vi "Reset Progress.vi"(8 "error in (no error)":errorcluster {"code" format="Error %.0f"}, 11 "UI Interaction in":refnum<class "UI Interaction.lvclass">) -> (0 "error out":errorcluster {"code" format="Error %.0f"}, 3 "UI Interaction out":refnum<class "UI Interaction.lvclass">)   [LabVIEW 2023, in "UI Interaction.lvclass"]
uses:
  UI Interaction.lvclass
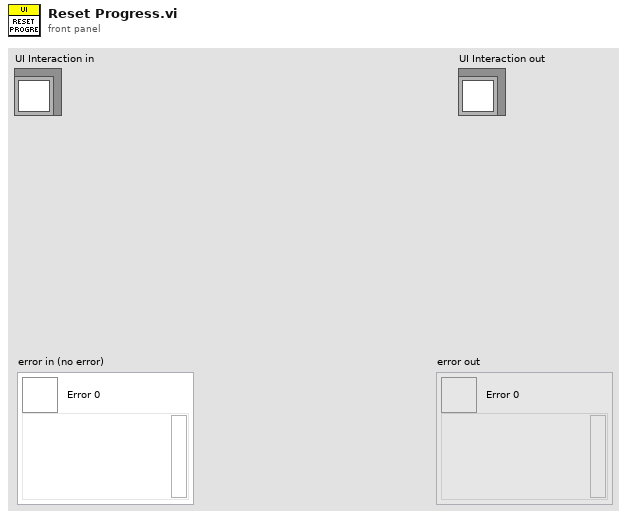
[diagram p1: front panel]
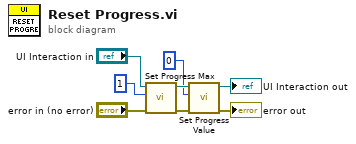
[diagram p0: block diagram]
diagram:
  n1 = call-dynamic "Set Progress Max.vi"("error in (no error)"="error in (no error)", "Progress Max"=1, "UI Interaction in"="UI Interaction in") -> ("error out"=w3:errorcluster, "UI Interaction out"=w8:refnum<class "UI Interaction.lvclass">)  [unwired: 7 in]
  n2 = call-dynamic "Set Progress Value.vi"("error in (no error)"=w3, "Progress Value"=0, "UI Interaction in"=w8) -> ("error out"=→"error out":errorcluster, "UI Interaction out"=→"UI Interaction out":refnum<class "UI Interaction.lvclass">)  [unwired: 7 in]
